vi "dfd_Super Narrowband Filter Design Shaping Filter Design.vi"(7 "filter type":T1(ring), 8 "error in (no error)":errorcluster, 9 "Shaping ripple specs":T7={"passband"=0.0, "stopband"=0.0, "dB/linear? (T: dB)"=TRUE}, 10 "Shaping freq specs [Hz]":T8, 11 "M":i32) -> (0 "error out":errorcluster, 3 "Shaping filter":T2={"mMRate_Structure"=enum."CIC", "mMRate_Mode"=0, "mMRate_Factor"=1, "mMRate_FIRParams"={"mMRate_FIR_H"=[], "mMRate_FIR_IsNyquist?"=FALSE, "mMRate_FIR_IsSymmetric?"=FALSE}, "mMRate_CICParams"={"mMRate_CIC_#Stage"=2, "mMRate_CIC_Lag"=1, "mMRate_CIC_Type"=enum."Lowpass"}, "mMRate_Order"=1, "mMRate_Version"="1.0", "mMRate_Comments"="1.0", "mMRate_RationalFactor"={"mMRate_L"=-1, "mMRate_M"=-1}, "mMRate_Fs"=1.0, "mMRate_Quantized?"=FALSE, "mMRate_QFilterGain"=1.0, "mMRate_CoefWl"=16, "mMRate_Scaling"={"mMRate_ScaleByPowerOf2?"=FALSE, "mMRate_ScaleType"=enum."Time Domain 1-Norm"}, "mMRate_InputWl"=0, "mMRate_OutputWl"=0, "mMRate_OutputMode"=enum."Nearest", "mMRate_MultMode"=enum."Truncated", "mMRate_BitPruning"=FALSE, "mMRate_GainWl"=16, "mMRate_OutputFwl"=0, "mMRate_SumIwl"=0, "mMRate_InputIwl "=16, "mMRate_SumWl"=32, "mMRate_CoefIwl"=0} {"mMRate_SumWl" min=1 max=32 step=1; "mMRate_InputIwl" min=1 max=32 step=1; "mMRate_GainWl" min=1 max=32 step=1; "mMRate_OutputWl" min=1 max=32 step=1; "mMRate_InputWl" min=1 max=32 step=1; "mMRate_CoefWl" min=1 max=32 step=1; "mMRate_Mode" items=["Default"=-1, "No Rate Change"=0, "Interpolation"=1, "Decimation"=2, "Interpolated"=3, "Rational"=4]})   [LabVIEW 2017, in "NI_DigFilter_Process.lvlib"]
uses:
  <vilib>/addons/Digital Filter Design/NI_DigFilter_Process.lvlib
  <vilib>/addons/Digital Filter Design/_Objects.llb/DFD Filter Frequence Specification (Design).ctl
  <vilib>/addons/Digital Filter Design/_Objects.llb/DFD Filter Ripple Specification (Design).ctl
  <vilib>/addons/Digital Filter Design/_Objects.llb/DFD Multirate Filter Obj.ctl
  <vilib>/addons/Digital Filter Design/_Objects.llb/DFD Multirate Mode.ctl
  <vilib>/addons/Digital Filter Design/_Objects.llb/DFD Coef Norm Type.ctl
  <vilib>/addons/Digital Filter Design/_Objects.llb/DFD Round-off Mode.ctl
  <vilib>/addons/Digital Filter Design/_Objects.llb/DFD FXP MRate Multiply Mode.ctl
  <vilib>/addons/Digital Filter Design/_REMEZ.llb/remez_fir filter type.ctl
  <vilib>/addons/Digital Filter Design/NI_DigFilterLicensed.lvlib
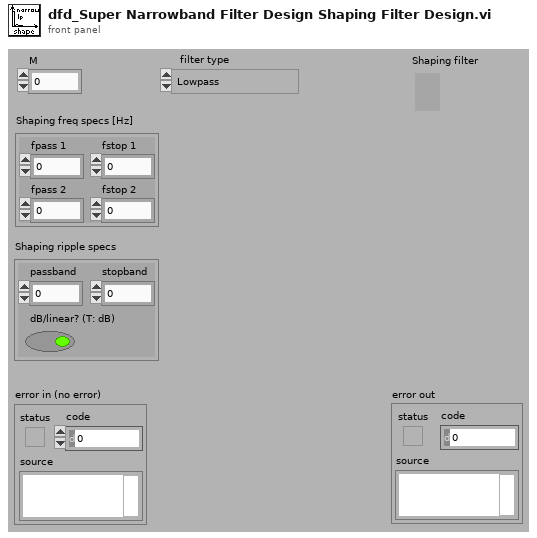
[diagram p1: front panel]
types:
  T1 = enum32{"Lowpass", "Highpass", "Bandpass", "Bandstop", "Wideband-Lowpass", "Wideband-Highpass"}
  T2 = typedef "NI_DigFilterLicensed.lvlib/DFD Multirate Filter Obj.ctl" = cluster{"mMRate_Structure":enum16{"CIC", "FIR", "IIR", "Lattice"}, "mMRate_Mode":T3, "mMRate_Factor":i32, "mMRate_FIRParams":cluster{"mMRate_FIR_H":dbl[], "mMRate_FIR_IsNyquist?":bool, "mMRate_FIR_IsSymmetric?":bool}, "mMRate_CICParams":cluster{"mMRate_CIC_#Stage":i32, "mMRate_CIC_Lag":i32, "mMRate_CIC_Type":enum16{"Lowpass", "Highpass"}}, "mMRate_Order":i32, "mMRate_Version":string, "mMRate_Comments":string, "mMRate_RationalFactor":cluster{"mMRate_L":i32, "mMRate_M":i32}, "mMRate_Fs":dbl, "mMRate_Quantized?":bool, "mMRate_QFilterGain":dbl, "mMRate_CoefWl":i16, "mMRate_Scaling":cluster{"mMRate_ScaleByPowerOf2?":bool, "mMRate_ScaleType":T4}, "mMRate_InputWl":i16, "mMRate_OutputWl":i16, "mMRate_OutputMode":T5, "mMRate_MultMode":T6, "mMRate_BitPruning":bool, "mMRate_GainWl":i16, "mMRate_OutputFwl":i16, "mMRate_SumIwl":i16, "mMRate_InputIwl ":i16, "mMRate_SumWl":i16, "mMRate_CoefIwl":i16}
  T3 = typedef "NI_DigFilterLicensed.lvlib/DFD Multirate Mode.ctl" = i16
  T4 = typedef "NI_DigFilterLicensed.lvlib/DFD Coef Norm Type.ctl" = enum16{"No Norm", "Time Domain 1-Norm", "Time Domain 2-Norm", "Time Domain Inf-Norm"}
  T5 = typedef "NI_DigFilterLicensed.lvlib/DFD Round-off Mode.ctl" = enum16{"Nearest", "Truncation"}
  T6 = typedef "NI_DigFilterLicensed.lvlib/DFD FXP MRate Multiply Mode.ctl" = enum16{"Truncated", "Full"}
  T7 = typedef "NI_DigFilterLicensed.lvlib/DFD Filter Ripple Specification (Design).ctl" = cluster{"passband":dbl, "stopband":dbl, "dB/linear? (T: dB)":bool}
  T8 = typedef "NI_DigFilterLicensed.lvlib/DFD Filter Frequence Specification (Design).ctl" = cluster{"fpass 1":dbl, "fstop 1":dbl, "fpass 2 ":dbl, "fstop 2":dbl}
  T9 = typedef "NI_DigFilterLicensed.lvlib/remez_fir filter type.ctl" = enum32{"Symmetric", "Antisymmetric", "Differentiator", "Hilbert", "Minimum Phase", "Maximum Phase"}
  T10 = typedef "NI_DigFilterLicensed.lvlib/DFD Adv Band Spec.ctl" = cluster{"band specification":cluster{"freq":dbl, "amplitude":dbl, "weight":dbl}[], "ripple constraint":dbl}
  T11 = typedef "NI_DigFilterLicensed.lvlib/DFD Filter Obj.ctl" = cluster{"mSRate_Fs":dbl, "mSRate_Version":string, "mSRate_Comments":string, "mSRate_OrgCoef":T12, "mSRate_CurCoef":T12, "mSRate_Quantized?":bool, "mSRate_QCoef":T12, "mSRate_QSettings":T14[], "mSRate_Order":i32, "mSRate_Scaling":cluster{"mSRate_ScaleByPowerOf2?":bool, "mSRate_ScaleType":T4}}
  T12 = typedef "NI_DigFilterLicensed.lvlib/DFD Filter Coef.ctl" = cluster{"type":T13, "gain":dbl, "coef a (k)":dbl[], "coef b (v)":dbl[]}
  T13 = typedef "NI_DigFilterLicensed.lvlib/DFD Filter Structure Type Selector.ctl" = enum16{"Undefined", "FIR Direct Form", "FIR Direct Form Transposed", "FIR Symmetric", "FIR Antisymmetric", "IIR Direct Form I", "IIR Direct Form I Transposed", "IIR Direct Form II", "IIR Direct Form II Transposed", "IIR Cascaded Second Order Sections Form I", "IIR Cascaded Second Order Sections Form I Transposed", "IIR Cascaded Second Order Sections Form II", "IIR Cascaded Second Order Sections Form II Transposed", "Lattice Allpass (basic sections)", "Lattice Allpass (one multiplier sections)", "Lattice Allpass (normalized sections)", "Lattice AR (basic sections)", "Lattice AR (one multiplier sections)", "Lattice AR (normalized sections)", "Lattice MA (minimum phase)", "Lattice MA (maximum phase)", "Lattice ARMA (basic sections)", "Lattice ARMA (one multiplier sections)", "Lattice ARMA (normalized sections)"}
  T14 = typedef "NI_DigFilterLicensed.lvlib/dfd_Internal Quantization Settings.ctl" = cluster{"source":T15, "wl":i16, "iwl":i16, "overflow mode":enum16{"Saturation", "Wrap"}, "rounding mode":enum16{"Nearest", "Truncation"}, "signed?":bool}
  T15 = typedef "NI_DigFilterLicensed.lvlib/dfd_Internal Quantization Srcs.ctl" = u16
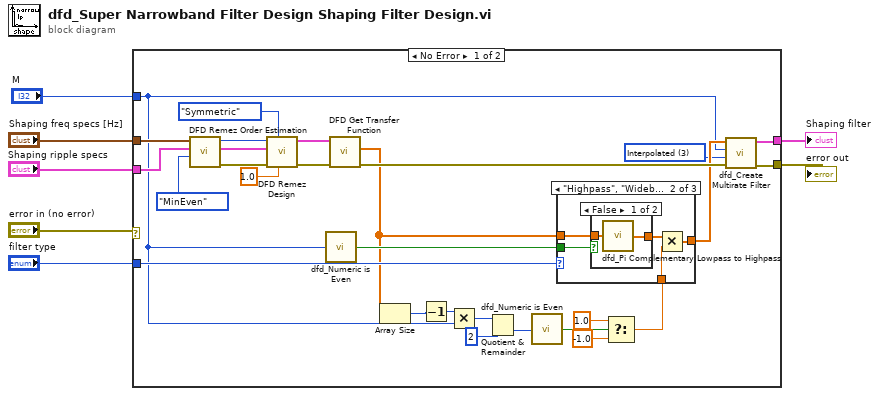
[diagram p0: block diagram]
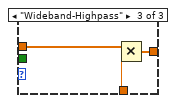
[diagram p4: hidden frame]
diagram:
  n1 = case shown="No Error" "error in (no error)" {
    selector: "error in (no error)" -> [_ w48]
    tunnel: "Shaping ripple specs" -> [w35 _]
    tunnel: "Shaping freq specs [Hz]" -> [w31 _]
    tunnel: "M" -> [w9 _]
    tunnel: "filter type" -> [w27 _]
    tunnel: [w12 _] -> w3
    tunnel: [w11 w48] -> w2
    frame No Error {
      w8 = T3 3 items=["Default"=-1, "No Rate Change"=0, "Interpolation"=1, "Decimation"=2, "Interpolated"=3] ("mode")
      n2 = call <vilib>:"DFD Remez Order Estimation.vi"("order option"=enum16{"MinNum", "MinEven", "MinOdd"}."MinEven", "ripple specs"=w35, "freq specs [Hz]"=w31) -> ("error out"=w34:errorcluster, "band specs"=w33:T10[], "estimated order"=w13:i32)  [unwired: 3 in, 3 out]
      n3 = call <vilib>:"DFD Remez Design.vi"("fs [Hz]"=1.0, "filter type"=remez_fir_filter_type."Symmetric", "error in (no error)"=w34, "band specs"=w33, "order"=w13) -> ("error out"=w28:errorcluster, "filter out"=w32:T11)  [unwired: 2 in, 3 out]
      n4 = call <vilib>:"dfd_Numeric is Even.vi"("N"=w9) -> ("even ?"=w25:bool)
      n5 = call <vilib>:"DFD Get Transfer Function.vi"("error in (no error)"=w28, "filter in"=w32) -> ("error out"=w26:errorcluster, "numerator"=w23:dbl[])  [unwired: 8 out]
      n6 = Array Size(array=w23) -> (size(s)=w22:i32)
      n7 = Decrement(x=w22) -> (x-1=w21:i32)
      n8 = Multiply(x=w21, y=w9) -> (x*y=w14:i32)
      n9 = Quotient & Remainder(x=w14, y=2) -> (floor(x/y)=w19:i32)  [unwired: 1 out]
      n10 = call <vilib>:"dfd_Numeric is Even.vi"("N"=w19) -> ("even ?"=w18:bool)
      n11 = Select(t=1.0, s=w18, f=-1.0) -> (s? t:f=w15:dbl)
      n12 = case shown="\"Highpass\", \"Wideband-Lowpass\"" w27 {
        tunnel: w23 -> [w36 w41 w46]
        tunnel: [w36 w38 w47] -> w10
        tunnel: w25 -> [_ w39 _]
        tunnel: w15 -> [_ w37 w45]
        frame "Lowpass", Default {
        }
        frame "Highpass", "Wideband-Lowpass" {
          n13 = case shown="False" w39 {
            tunnel: w41 -> [w43 w44]
            tunnel: [w42 w44] -> w40
            frame False {
              n14 = call <vilib>:"dfd_Pi Complementary Lowpass to Highpass.vi"("Lowpass"=w43) -> ("Highpass"=w42:dbl[])
            }
            frame True {
            }
          }
          n15 = Multiply(x=w40, y=w37) -> (x*y=w38:dbl[])
        }
        frame "Wideband-Highpass" {
          n16 = Multiply(x=w46, y=w45) -> (x*y=w47:dbl[])
        }
      }
      n17 = call <vilib>:"dfd_Create Multirate Filter.vi"("error in (no error)"=w26, "mode"=w8, "factor"=w9, "h (n)"=w10) -> ("error out"=w11:errorcluster, "multirate filter out"=w12:T2)  [unwired: 1 in, 5 out]
    }
    frame Error {
    }
  }
  "error out" <- w2
  "Shaping filter" <- w3
